vi "stopmeas.vi"() -> ()   [LabVIEW 2019]
panel:
  out "error out":errorcluster
  out "ctcstatus":i32
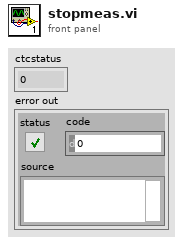
[diagram p1: front panel]
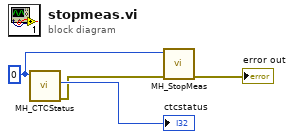
[diagram p0: block diagram]
diagram:
  w1 = 0 ("devidx")
  n1 = call <userlib>:"MH_CTCStatus.vi"("devidx"=w1) -> ("error out"=w3:errorcluster, "ctcstatus"=→"ctcstatus":i32)  [unwired: 8 in, 1 out]
  n2 = call <userlib>:"MH_StopMeas.vi"("error in (no error)"=w3, "devidx"=w1) -> ("error out"=→"error out":errorcluster)  [unwired: 8 in, 1 out]
